vi "BNC2090 q meter.vi"() -> ()   [LabVIEW 2009]
panel:
  in  "stop (F) 2":bool caption="stop (F)"
  out "Waveform Graph 2":dynamicdata(graph)
  out "Waveform Graph":dynamicdata(graph)
  in  "stop (F)":bool
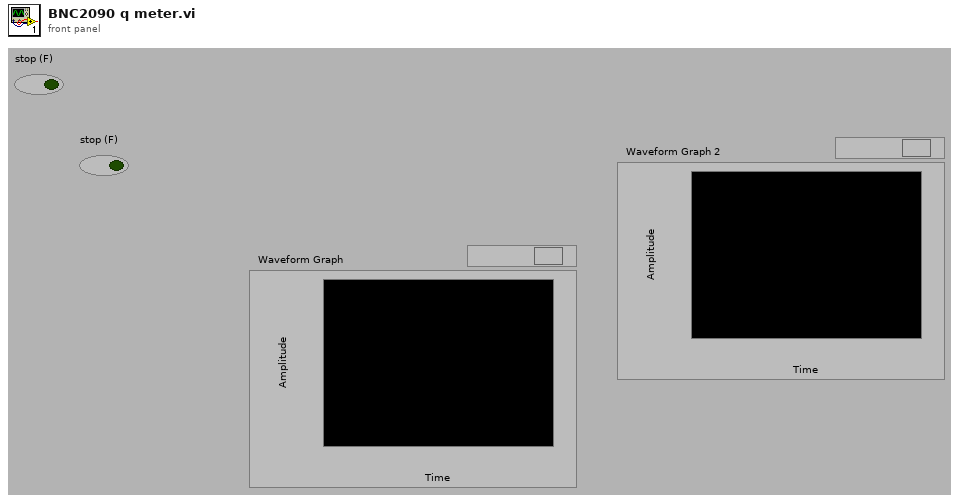
[diagram p1: front panel]
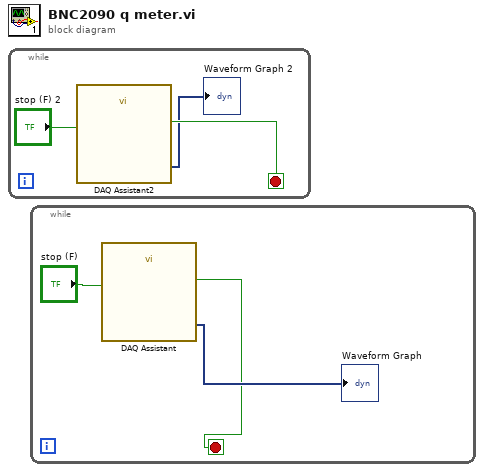
[diagram p0: block diagram]
diagram:
  n1 = while {
    stop <- w2 stop-if-true
    n2 = call "DAQ Assistant2"("stop (F)"="stop (F) 2") -> ("data"=→"Waveform Graph 2":dynamicdata, "stopped"=w2:bool)  [unwired: 15 in, 2 out]
  }
  n3 = while {
    stop <- w5 stop-if-true
    n4 = call "DAQ Assistant"("stop (F)"="stop (F)") -> ("data"=→"Waveform Graph":dynamicdata, "stopped"=w5:bool)  [unwired: 15 in, 2 out]
  }
